vi "Test-Forward Drive.vi"() -> ()   [LabVIEW 2014, in "Comp Driver.lvlib"]
uses:
  Comp Driver.lvlib
  Robot Actor Framework/Trace/Trace Controller Class/Config.ctl
  Comp Motors with Encoders/Comp Motors with Encoders Class/Motor Controller Config.ctl
  Robot/Motor with Encoders/Motors with Encoders Class/Motors with Encoders Config.ctl
  Comp Motors with Encoders/Comp Motors with Encoders Class/Encoder Config.ctl
  Robot/Forward Drive/Forward Drive Class/Forward Drive Config.ctl
  Robot/Motor with Encoders/Motors with Encoders Class/Motors with Encoders.lvclass
  Comp Trace Controller/Comp Trace Controller Class/Comp Trace Controller.lvclass
  Comp Pressure/Comp Pressure Class/Comp Pressure.lvclass
  Robot/Forward Drive/Forward Drive Class/Forward Drive.lvclass
  Comp Motors with Encoders/Comp Motors with Encoders Class/Comp Motors with Encoders.lvclass
  <vilib>/Rock Robotics/WPI/DriverStation/WPI_DriverStationRobotMode2.ctl
  Robot/Forward Drive/Forward Drive Messages/Set Percentage Msg/Set Percentage Msg.lvclass/Set Percentage Msg.ctl
  <vilib>/ActorFramework/Message Enqueuer/Message Enqueuer.lvclass/Message Enqueuer.ctl
  <vilib>/ActorFramework/Message Enqueuer/Enqueue.vi
  <vilib>/ActorFramework/Message Priority Queue/Priority Enqueue.vi
  Robot/Forward Drive/Forward Drive Messages/Set Percentage Msg/Set Percentage Msg.lvclass
  <vilib>/ActorFramework/Stop Msg/Stop Msg.lvclass
  <vilib>/ActorFramework/Actor/Actor.lvclass
  Robot Actor Framework/Trace/Trace Controller Class/Trace Controller.lvclass
panel:
  in  "Test Loop":u32=50
  in  "Right Encoder Config":T1={"P"=1.0, "D"=0.0, "F"=0.01, "I"=0.01, "Reverse Feedback Sensor"=TRUE, "Encoder Codes Per Rev"=256}
  in  "Right Slaves":T2[](array[typedef])=[{"Device Number"=5, "Invert Motor"=FALSE}]
  in  "Right Master":T2={"Device Number"=4, "Invert Motor"=TRUE}
  in  "Right":dbl(slide)=0.02040816326530604 scale=-1.0..1.0
  in  "Forward Drive Config":T3={"Left Motors with Encoders"=refnum, "Right Motors with Encoders"=refnum, "Encoder Control"=TRUE}
  in  "Left Encoder Config":T1={"P"=1.0, "D"=0.0, "F"=0.01, "I"=0.01, "Reverse Feedback Sensor"=TRUE, "Encoder Codes Per Rev"=256}
  out "Enable Tele":bool caption="Enabled Teleop"
  in  "Stop Test Loop 1":bool=TRUE
  in  "Finish Test":bool=TRUE
  in  "Start Test":bool=TRUE
  in  "Left":dbl(slide)=0.02040816326530604 scale=-1.0..1.0
  in  "Motors with Encoder Config":T4={"Counts  Per Revolution"=256, "Invert Encoder Direction"=FALSE, "Diameter of Revolution"=6.0, "Max RPM"=1900.0, "Encoder Control"=TRUE}
  in  "Left Slave Motor Controller Configs":T2[](array[typedef])=[{"Device Number"=10, "Invert Motor"=FALSE}]
  in  "left Master Motor Controller Config":T2={"Device Number"=9, "Invert Motor"=FALSE}
  in  "Config":T5={"Folder Pattern"="/media/sd%s1", "Starting Letter Position"=1, "Min Free Space (MB)"=50.0, "Max Folders to Check"=10, "Trace Level"=enum."Debug"} {"Min Free Space (MB)" format="%#_13g"}
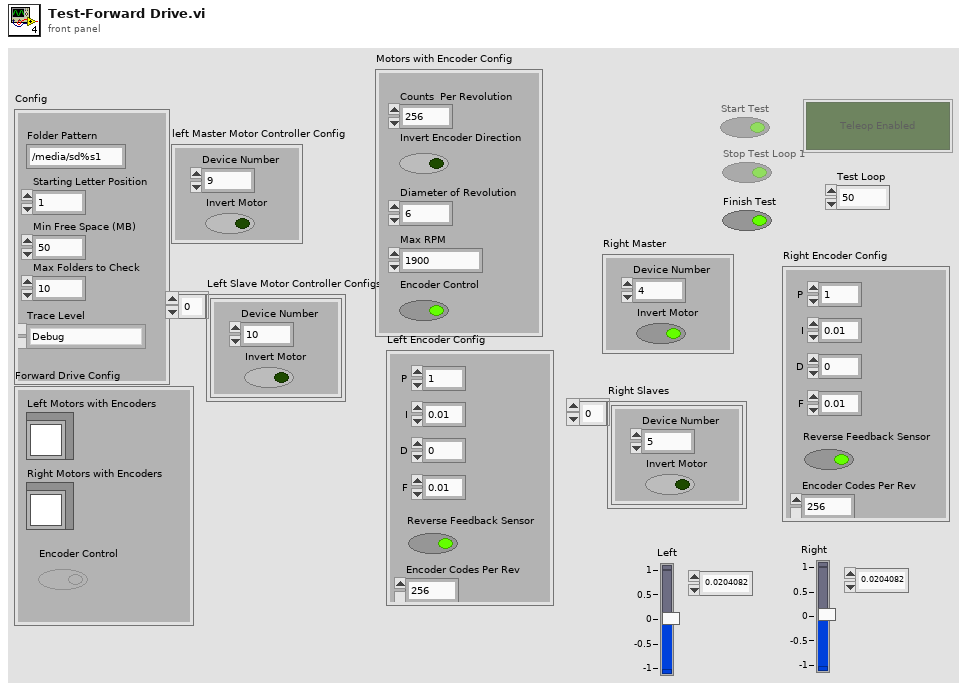
[diagram p1: front panel]
types:
  T1 = typedef "Comp Motors with Encoders.lvlib/Comp Motors with Encoders.lvclass/Encoder Config.ctl" = cluster{"P":dbl, "D":dbl, "F":dbl, "I":dbl, "Reverse Feedback Sensor":bool, "Encoder Codes Per Rev":u16}
  T2 = typedef "Comp Motors with Encoders.lvlib/Comp Motors with Encoders.lvclass/Motor Controller Config.ctl" = cluster{"Device Number":u8, "Invert Motor":bool}
  T3 = typedef "Forward Drive.lvlib/Forward Drive.lvclass/Forward Drive Config.ctl" = cluster{"Left Motors with Encoders":refnum<class "Motors with Encoders.lvclass">, "Right Motors with Encoders":refnum<class "Motors with Encoders.lvclass">, "Encoder Control":bool}
  T4 = typedef "Motors with Encoders.lvlib/Motors with Encoders.lvclass/Motors with Encoders Config.ctl" = cluster{"Counts  Per Revolution":u32, "Invert Encoder Direction":bool, "Diameter of Revolution":dbl, "Max RPM":dbl, "Encoder Control":bool}
  T5 = typedef "Robot Actor Framework.lvlib/Trace.lvlib/Trace Controller.lvclass/Config.ctl" = cluster{"Folder Pattern":string, "Starting Letter Position":i32, "Min Free Space (MB)":dbl, "Max Folders to Check":u32, "Trace Level":enum16{"Critical", "Error", "Warning", "Informational", "Debug"}}
  T6 = enum16{"Critical", "Error", "Warning", "Informational", "Debug"}
  T7 = enum8{"Enabled", "Disabled", "Disabled and Grayed Out"}
  T8 = typedef "WPI_DriverStationRobotMode2.ctl" = enum16{"Autonomous Disabled", "Autonomous Enabled", "Teleop Disabled", "Teleop Enabled", "Disconnected", "Finish", "Test Disabled", "Test Enabled", "Emergency Stopped"}
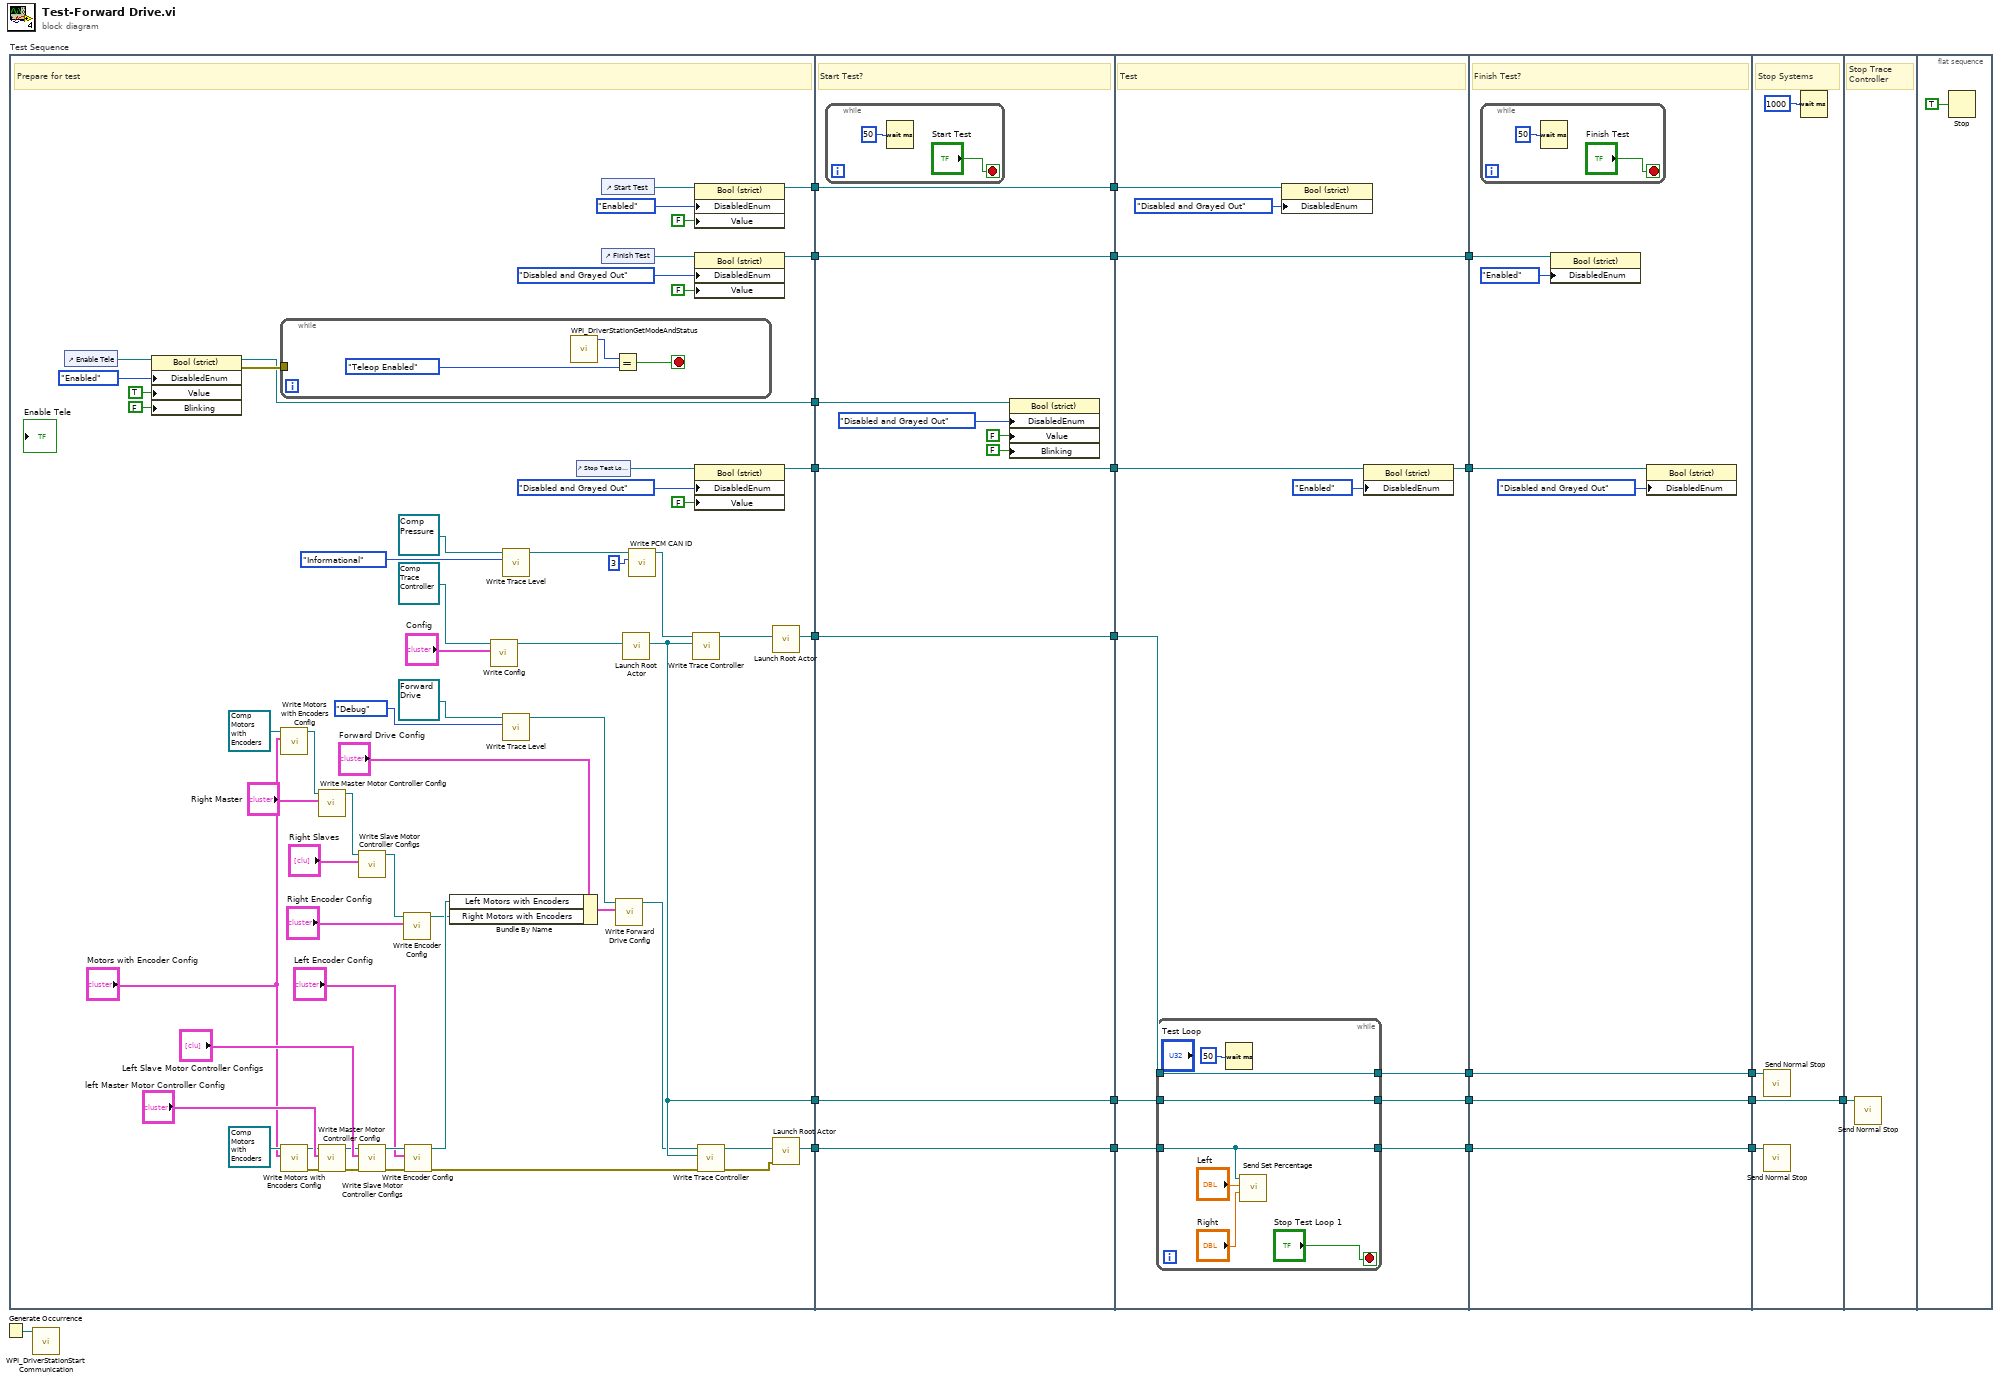
[diagram p0: block diagram]
diagram:
  n1 = Generate Occurrence() -> (w23:refnum<k4>)
  n2 = flat-sequence "Test Sequence" {
    tunnel: [w43] -> w12
    tunnel: [w66] -> w11
    tunnel: [w65] -> w10
    tunnel: [w55] -> w9
    tunnel: [w54] -> w7
    tunnel: [w53] -> w2
    tunnel: [w47] -> w1
    tunnel: [w95] -> w15
    tunnel: [w94] -> w14
    tunnel: [w93] -> w13
    tunnel: w12 -> [w95]
    tunnel: w11 -> [w94]
    tunnel: w10 -> [w93]
    tunnel: w9 -> [w92]
    tunnel: [w92] -> w8
    tunnel: w7 -> [w91]
    tunnel: [w91] -> w6
    tunnel: [w90] -> w3
    tunnel: w2 -> [w90]
    tunnel: w1 -> [w89]
    tunnel: [w104] -> w18
    tunnel: [w106] -> w17
    tunnel: [w105] -> w16
    tunnel: w15 -> [w109]
    tunnel: w14 -> [w107]
    tunnel: w13 -> [w108]
    tunnel: w8 -> [w103]
    tunnel: w6 -> [w101]
    tunnel: [w99] -> w5
    tunnel: [w98] -> w4
    tunnel: w3 -> [w98]
    tunnel: [w123] -> w21
    tunnel: [w122] -> w20
    tunnel: [w121] -> w19
    tunnel: w18 -> [w123]
    tunnel: w17 -> [w122]
    tunnel: w16 -> [w121]
    tunnel: w5 -> [w120]
    tunnel: w4 -> [w117]
    tunnel: [w129] -> w22
    tunnel: w21 -> [w129]
    tunnel: w20 -> [w128]
    tunnel: w19 -> [w126]
    tunnel: w22 -> [w130]
    frame #0 {
      # "Prepare for test"
      n3 = control-ref of="Enable Tele"() -> (w52:refnum<vi>)
      n4 = property class="Bool (strict)"(reference=w52, "DisabledEnum"=T7."Enabled" ("Disabled"), "Value"=TRUE, "Blinking"=FALSE) -> (reference out=w47:refnum<vi>, error out=w49:errorcluster)  [unwired: 1 in]
      n5 = while {
        tunnel: w49 -> [_]
        stop <- w83 stop-if-true
        n6 = call <vilib>:"WPI_DriverStationGetModeAndStatus.vi"() -> ("Robot Mode"=w85:T8)  [unwired: 10 in, 1 out]
        n7 = Equal?(x=w85, y=WPI_DriverStationRobotMode2."Teleop Enabled") -> (x = y?=w83:bool)
      }
      n8 = call-dynamic "Write Motors with Encoders Config.vi"("Motors with Encoders Config"="Motors with Encoder Config", "Motors with Encoders in"=refnum<class "Comp Motors with Encoders.lvclass"> refnum ("Comp Motors with Encoders.lvlib:Comp Motors with Encoders.lvclass")) -> ("Motors with Encoders out"=w32:refnum<class "Comp Motors with Encoders.lvclass">)  [unwired: 8 in, 1 out]
      n9 = call-dynamic "Write Motors with Encoders Config.vi"("Motors with Encoders Config"="Motors with Encoder Config", "Motors with Encoders in"=refnum<class "Comp Motors with Encoders.lvclass"> refnum ("Comp Motors with Encoders.lvlib:Comp Motors with Encoders.lvclass")) -> ("error out"=w73:errorcluster, "Motors with Encoders out"=w34:refnum<class "Comp Motors with Encoders.lvclass">)  [unwired: 8 in]
      n10 = call-dynamic "Write Master Motor Controller Config.vi"("Master Motor Controller Config"="Right Master", "Comp Motors with Encoders in"=w32) -> ("Comp Motors with Encoders out"=w31:refnum<class "Comp Motors with Encoders.lvclass">)  [unwired: 8 in, 1 out]
      n11 = call-dynamic "Write Master Motor Controller Config.vi"("error in (no error)"=w73, "Master Motor Controller Config"="left Master Motor Controller Config", "Comp Motors with Encoders in"=w34) -> ("error out"=w74:errorcluster, "Comp Motors with Encoders out"=w70:refnum<class "Comp Motors with Encoders.lvclass">)  [unwired: 7 in]
      n12 = call-dynamic "Write Slave Motor Controller Configs.vi"("Slave Motor Controller Configs"="Right Slaves", "Comp Motors with Encoders in"=w31) -> ("Comp Motors with Encoders out"=w30:refnum<class "Comp Motors with Encoders.lvclass">)  [unwired: 8 in, 1 out]
      n13 = call-dynamic "Write Slave Motor Controller Configs.vi"("error in (no error)"=w74, "Slave Motor Controller Configs"="Left Slave Motor Controller Configs", "Comp Motors with Encoders in"=w70) -> ("error out"=w45:errorcluster, "Comp Motors with Encoders out"=w46:refnum<class "Comp Motors with Encoders.lvclass">)  [unwired: 7 in]
      n14 = call-dynamic "Write Encoder Config.vi"("Encoder Config"="Right Encoder Config", "Comp Motors with Encoders in"=w30) -> ("Comp Motors with Encoders out"=w29:refnum<class "Comp Motors with Encoders.lvclass">)  [unwired: 8 in, 1 out]
      n15 = call-dynamic "Write Encoder Config.vi"("error in (no error)"=w45, "Encoder Config"="Left Encoder Config", "Comp Motors with Encoders in"=w46) -> ("error out"=w44:errorcluster, "Comp Motors with Encoders out"=w40:refnum<class "Comp Motors with Encoders.lvclass">)  [unwired: 7 in]
      n16 = Bundle By Name(cluster="Forward Drive Config", "Left Motors with Encoders"=w40, "Right Motors with Encoders"=w29) -> (w41:T3)
      n17 = call-dynamic "Write Config.vi"("Config"="Config", "Trace Controller in"=refnum<class "Comp Trace Controller.lvclass"> refnum ("Comp Trace Controller.lvlib:Comp Trace Controller.lvclass")) -> ("Trace Controller out"=w69:refnum<class "Comp Trace Controller.lvclass">)  [unwired: 8 in, 1 out]
      n18 = call-dynamic "Write Trace Level.vi"("Trace Level"=T6."Informational", "System Actor in"=refnum<class "Comp Pressure.lvclass"> refnum ("Comp Pressure.lvlib:Comp Pressure.lvclass")) -> ("System Actor out"=w79:refnum<class "Comp Pressure.lvclass">)  [unwired: 8 in, 1 out]
      n19 = call-dynamic "Write Trace Level.vi"("Trace Level"=T6."Debug", "System Actor in"=refnum<class "Forward Drive.lvclass"> refnum ("Forward Drive.lvlib:Forward Drive.lvclass")) -> ("System Actor out"=w37:refnum<class "Forward Drive.lvclass">)  [unwired: 8 in, 1 out]
      n20 = control-ref of="Stop Test Loop 1"() -> (w59:refnum<vi>)
      n21 = control-ref of="Start Test"() -> (w64:refnum<vi>)
      n22 = control-ref of="Finish Test"() -> (w58:refnum<vi>)
      n23 = call-dynamic "Write Forward Drive Config.vi"("Forward Drive Config"=w41, "Forward Drive in"=w37) -> ("Forward Drive out"=w39:refnum<class "Forward Drive.lvclass">)  [unwired: 8 in, 1 out]
      n24 = call <vilib>:"Launch Root Actor.vi"("Actor"=w69) -> ("Actor's Enqueuer"=w65:refnum<class "Message Enqueuer.lvclass">)  [unwired: 9 in, 1 out]
      n25 = call-dynamic "Write PCM CAN ID.vi"("PCM CAN ID"=u8 3, "Comp Pressure in"=w79) -> ("Comp Pressure out"=w81:refnum<class "Comp Pressure.lvclass">)  [unwired: 8 in, 1 out]
      n26 = call-dynamic "Write Trace Controller.vi"("Trace Controller"=w65, "System Actor in"=w81) -> ("System Actor out"=w82:refnum<class "Comp Pressure.lvclass">)  [unwired: 8 in, 1 out]
      n27 = property class="Bool (strict)"(reference=w64, "DisabledEnum"=T7."Enabled" ("Disabled"), "Value"=FALSE) -> (reference out=w55:refnum<vi>)  [unwired: 1 in, 1 out]
      n28 = property class="Bool (strict)"(reference=w58, "DisabledEnum"=T7."Disabled and Grayed Out" ("Disabled"), "Value"=FALSE) -> (reference out=w53:refnum<vi>)  [unwired: 1 in, 1 out]
      n29 = property class="Bool (strict)"(reference=w59, "DisabledEnum"=T7."Disabled and Grayed Out" ("Disabled"), "Value"=FALSE) -> (reference out=w54:refnum<vi>)  [unwired: 1 in, 1 out]
      n30 = call-dynamic "Write Trace Controller.vi"("error in (no error)"=w44, "Trace Controller"=w65, "System Actor in"=w39) -> ("error out"=w76:errorcluster, "System Actor out"=w75:refnum<class "Forward Drive.lvclass">)  [unwired: 7 in]
      n31 = call <vilib>:"Launch Root Actor.vi"("Actor"=w82) -> ("Actor's Enqueuer"=w66:refnum<class "Message Enqueuer.lvclass">)  [unwired: 9 in, 1 out]
      n32 = call <vilib>:"Launch Root Actor.vi"("error in (no error)"=w76, "Actor"=w75) -> ("Actor's Enqueuer"=w43:refnum<class "Message Enqueuer.lvclass">)  [unwired: 8 in, 1 out]
    }
    frame #1 {
      # "Start Test?"
      n33 = while {
        stop <- "Start Test" stop-if-true
        n34 = Wait (ms)(milliseconds to wait=u32 50) -> ()  [unwired: 1 out]
      }
      n35 = property class="Bool (strict)"(reference=w89, "DisabledEnum"=T7."Disabled and Grayed Out" ("Disabled"), "Value"=FALSE, "Blinking"=FALSE) -> ()  [unwired: 1 in, 2 out]
    }
    frame #2 {
      # "Test"
      n36 = while {
        tunnel: w108 -> [w115]
        tunnel: [w115] -> w104
        tunnel: w109 -> [w112]
        tunnel: [w112] -> w106
        tunnel: w107 -> [w114]
        tunnel: [w114] -> w105
        stop <- "Stop Test Loop 1" stop-if-true
        n37 = Wait (ms)(milliseconds to wait=u32 50) -> ()  [unwired: 1 out]
        n38 = call "Send Set Percentage.vi"("Right Percentage"="Right", "Left Percentage"="Left", "Message Enqueuer"=w112) -> ()  [unwired: 7 in, 2 out]
      }
      n39 = property class="Bool (strict)"(reference=w103, "DisabledEnum"=T7."Disabled and Grayed Out" ("Disabled")) -> ()  [unwired: 1 in, 2 out]
      n40 = property class="Bool (strict)"(reference=w101, "DisabledEnum"=T7."Enabled" ("Disabled")) -> (reference out=w99:refnum<vi>)  [unwired: 1 in, 1 out]
    }
    frame #3 {
      # "Finish Test?"
      n41 = while {
        stop <- "Finish Test" stop-if-true
        n42 = Wait (ms)(milliseconds to wait=u32 50) -> ()  [unwired: 1 out]
      }
      n43 = property class="Bool (strict)"(reference=w117, "DisabledEnum"=T7."Enabled" ("Disabled")) -> ()  [unwired: 1 in, 2 out]
      n44 = property class="Bool (strict)"(reference=w120, "DisabledEnum"=T7."Disabled and Grayed Out" ("Disabled")) -> ()  [unwired: 1 in, 2 out]
    }
    frame #4 {
      # "Stop Systems"
      n45 = call <vilib>:"Send Normal Stop.vi"("Message Enqueuer"=w126) -> ()  [unwired: 10 in, 1 out]
      n46 = call <vilib>:"Send Normal Stop.vi"("Message Enqueuer"=w128) -> ()  [unwired: 10 in, 1 out]
      n47 = Wait (ms)(milliseconds to wait=u32 1000) -> ()  [unwired: 1 out]
    }
    frame #5 {
      # "Stop Trace Controller"
      n48 = call <vilib>:"Send Normal Stop.vi"("Message Enqueuer"=w130) -> ()  [unwired: 10 in, 1 out]
    }
    frame #6 {
      n49 = Stop(stop? (T)=TRUE) -> ()
    }
  }
  n50 = call <vilib>:"WPI_DriverStationStart Communication.vi"("occurrence"=w23) -> ()  [unwired: 1 in, 10 out]
